vi "Convert ASCII String to Hex String.vi"(8 "error in":errorcluster, 11 "ASCII string in":string) -> (0 "error out":errorcluster, 3 "hex string out":string)   [LabVIEW 2011]
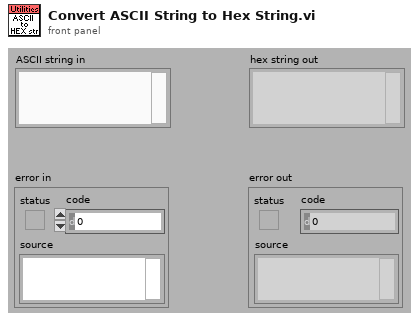
[diagram p1: front panel]
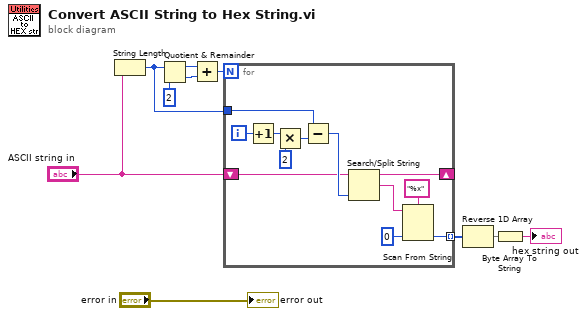
[diagram p0: block diagram]
diagram:
  n1 = String Length(string="ASCII string in") -> (length=w6:i32)
  n2 = Quotient & Remainder(x=w6, y=2) -> (x-y*floor(x/y)=w9:i32, floor(x/y)=w3:i32)
  n3 = Add(x=w9, y=w3) -> (x+y=w8:i32)
  n4 = for {
    N: w8 -> [_]
    tunnel: w6 -> [w19]
    tunnel: [w17] -> w5 mode=indexing
    shift-right: [w12] -> _
    shift-left: "ASCII string in" -> [w13]
    i -> [w21]
    n5 = Increment(x=w21) -> (x+1=w15:i32)
    n6 = Multiply(x=w15, y=2) -> (x*y=w16:i32)
    n7 = Subtract(x=w19, y=w16) -> (x-y=w22:i32)
    n8 = Search/Split String(string=w13, offset (0)=w22) -> (substring before match=w12:string, match + rest of string=w11:string)  [unwired: 2 out]
    n9 = Scan From String(format string="%x", input string=w11, default 1=u8 0 ("default value 1")) -> (output 1=w17:u8)  [unwired: 2 in, 3 out]
  }
  n10 = Reverse 1D Array(array=w5) -> (reversed array=w4:u8[])
  n11 = Byte Array To String(unsigned byte array=w4) -> (string=→"hex string out":string)
  "error out" <- "error in"
